vi "Teleop.vi"(10 "Match Info":T3={"Autonomous Elapsed Seconds"=0.0, "TeleOp Elapsed Seconds"=0.0, "Disabled Elapsed Seconds"=0.0, "Visited Autonomous"=FALSE, "Visited TeleOp"=FALSE, "Visited Disabled"=FALSE, "Autonomous Settings"={"Autonomous Style"=enum."Independent", "VI Refnum"=refnum}}, 11 "Call Context":T4) -> ()   [LabVIEW 2020]
doc: "This VI is called for each TeleOp packet received from the DS where the robot is not disabled. It is often used to read from the joysticks and update I/O or to update setpoints for timed control loops. It should complete and return within 20 milliseconds or it may miss DS packets."
uses:
  <vilib>/Rock Robotics/WPI/DriverStation/WPI_DriverStationDerivedRobotMode.ctl
  <vilib>/Rock Robotics/WPI/DriverStation/WPI_DriverStationMatch Info.ctl
  <vilib>/Rock Robotics/WPI/ThirdParty/Phoenix-LabVIEW/Motor Controller/Controls/CTRE_Phoenix_MotorControl_ControlMode.ctl
  <vilib>/Rock Robotics/WPI/Utilities/WPI_GetSetVariantRefNum.vi
  <vilib>/Rock Robotics/Network Tables/NT Write Boolean Array.vi
  <vilib>/Rock Robotics/Network Tables/NT Write Numeric Array.vi
  <vilib>/Rock Robotics/WPI/ThirdParty/Phoenix-LabVIEW/Motor Controller/Get/CTRE_Phoenix_MotorController_GetSelectedSensorData.vi
  <vilib>/Rock Robotics/WPI/ThirdParty/Phoenix-LabVIEW/Motor Controller/Get/CTRE_Phoenix_MotorController_GetSupplyAndStatorCurrent_Enhanced.vi
  TitanLib/Lib/TitanLib.lvlib
panel:
  in  "I Zone":dbl=1000.0
  in  "F":dbl=0.0461
  in  "D":dbl
  in  "I":dbl=0.001
  in  "P":dbl=0.1
  in  "Set PIDF":bool=TRUE
  in  "Setpoint":dbl=7000.0
  out "Current":T1(graph)
  out "PID Output":T2(graph)
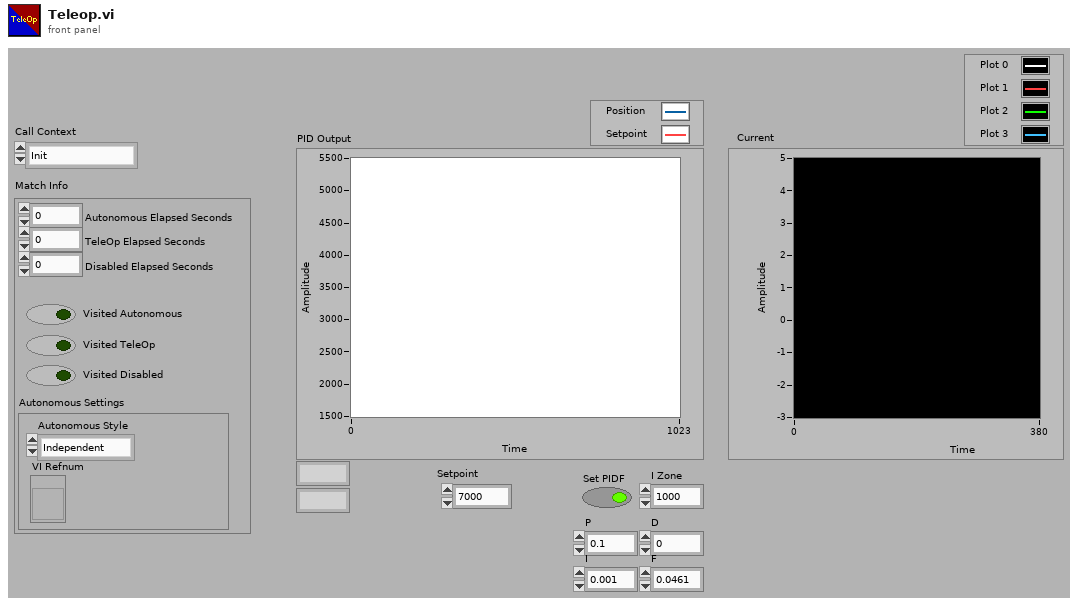
[diagram p1: front panel]
types:
  T1 = cluster{"Supply Current":dbl, "Stator Current":dbl}
  T2 = cluster{"Setpoint Position":dbl, "Position (Raw Sensor Units)":i32}
  T3 = typedef "WPI_DriverStationMatch Info.ctl" = cluster{"Autonomous Elapsed Seconds":dbl, "TeleOp Elapsed Seconds":dbl, "Disabled Elapsed Seconds":dbl, "Visited Autonomous":bool, "Visited TeleOp":bool, "Visited Disabled":bool, "Autonomous Settings":cluster{"Autonomous Style":enum16{"Iterative", "Independent"}, "VI Refnum":refnum<vi>}}
  T4 = typedef "WPI_DriverStationDerivedRobotMode.ctl" = enum16{"Init", "Execute", "Stop"}
  T5 = typedef "WPI_JoystickDevRef.ctl" = cluster{"Device":T6}
  T6 = typedef "WPI_JoystickDeviceEnum.ctl" = enum16{"USB 0", "USB 1", "USB 2", "USB 3", "USB 4", "USB 5"}
  T7 = typedef "WPI_MotorControlDeviceRef.ctl" = cluster{"DeviceStatus":errorcluster, "Type":T8, "PWM":cluster{"PWM Channel":T9, "DeadBand":T10}, "CAN":cluster{"Device Number":u8, "SetOutput VI Ref":variant, "GetOutput VI Ref":variant, "Enable VI Ref":variant, "Disable VI Ref":variant, "Data":variant}, "Invert":bool, "DIO PWM":cluster{"PWM \"Enable\" Channel":T9, "DIOChannel":T11, "PWM Rate":dbl}}
  T8 = typedef "WPI_MotorControlType.ctl" = enum16{"PWM", "CAN", "DIO PWM"}
  T9 = typedef "FPGA_DIOPWMChannel.ctl" = enum8{"PWM 0", "PWM 1", "PWM 2", "PWM 3", "PWM 4", "PWM 5", "PWM 6", "PWM 7", "PWM 8", "PWM 9", "PWM MXP 0", "PWM MXP 1", "PWM MXP 2", "PWM MXP 3", "PWM MXP 4", "PWM MXP 5", "PWM MXP 6", "PWM MXP 7", "PWM MXP 8", "PWM MXP 9", "Invalid"}
  T10 = typedef "WPI_PWMDeadband.ctl" = cluster{"Name":string, "maxPositivePwm":i32, "minPositivePwm":i32, "centerPwm":i32, "maxNegativePwm":i32, "minNegativePwm":i32, "angularRange":u16}
  T11 = typedef "FPGA_DIOChannel.ctl" = enum8{"DIO 0", "DIO 1", "DIO 2", "DIO 3", "DIO 4", "DIO 5", "DIO 6", "DIO 7", "DIO 8", "DIO 9", "DIO MXP 0", "DIO MXP 1", "DIO MXP 2", "DIO MXP 3", "DIO MXP 4", "DIO MXP 5", "DIO MXP 6", "DIO MXP 7", "DIO MXP 8", "DIO MXP 9", "DIO MXP 10", "DIO MXP 11", "DIO MXP 12", "DIO MXP 13", "DIO MXP 14", "DIO MXP 15", "SPI Port CS1", "SPI Port CS2", "SPI Port CS3", "SPI Port MISO", "SPI Port MOSI", "Invalid"}
  T12 = typedef "CTRE_Phoenix_MotorControl_ControlMode.ctl" = u16
  T13 = cluster{"Setpoint":dbl, "Position (Raw Sensor Units)":i32}
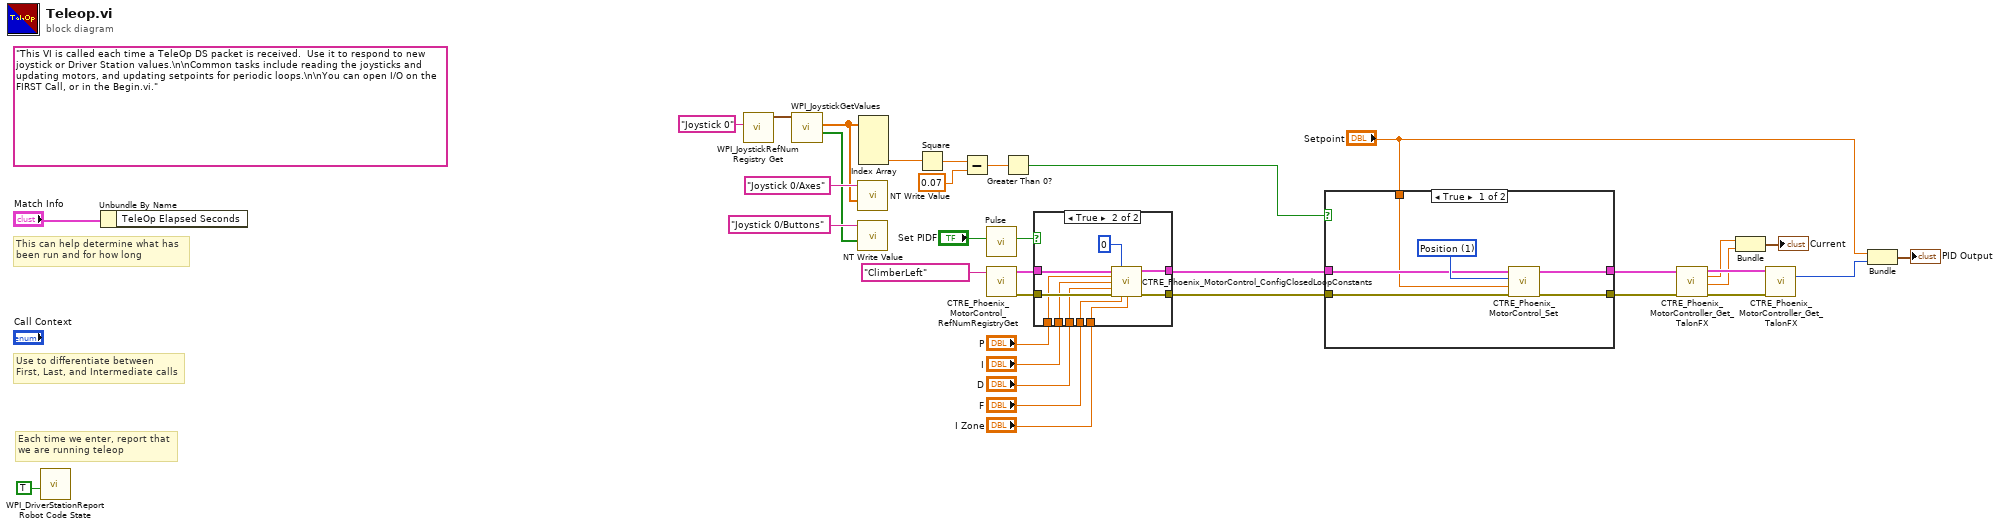
[diagram p0: block diagram]
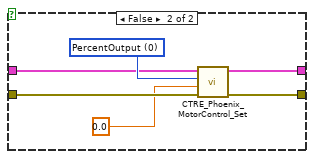
[diagram p2: hidden frame]
diagram:
  (unwired) "This VI is called each time a TeleOp DS packet is received.  Use it to respond to new joystick or Driver Station values.\n\nCommon tasks include reading the joysticks and updating motors, and updating setpoints for periodic loops.\n\nYou can open I/O on the FIRST Call, or in the Begin.vi."
  # "Each time we enter, report that\nwe are running teleop"
  # "Use to differentiate between\nFirst, Last, and Intermediate calls"
  # "This can help determine what has\nbeen run and for how long"
  n1 = call <vilib>:"WPI_DriverStationReport Robot Code State.vi"("TeleOp"=TRUE ("Autonomous")) -> ()  [unwired: 10 in, 1 out]
  n2 = Unbundle By Name("Match Info") -> ()  [unwired: 1 out]
  n3 = call <vilib>:"WPI_JoystickRefNum Registry Get.vi"("refnum name"="Joystick 0") -> ("JoystickDevRef"=w33:T5)  [unwired: 1 in, 9 out]
  n4 = call <vilib>:"WPI_JoystickGetValues.vi"("JoystickDevRef"=w33) -> ("Buttons"=w10:bool[], "Axes"=w29:dbl[])  [unwired: 6 in, 3 out]
  n5 = call-poly <vilib>:"NT Write Value.vi"("Numeric Array"=w29, "Name"="Joystick 0/Axes") -> ()  [unwired: 9 in, 1 out]
  n6 = call-poly <vilib>:"NT Write Value.vi"("Boolean Array"=w10, "Name"="Joystick 0/Buttons") -> ()  [unwired: 9 in, 1 out]
  n7 = Index Array(array=w29) -> (element #4=w4:dbl)  [unwired: 4 in, 3 out]
  n8 = Square(x=w4) -> (x^2=w8:dbl)
  n9 = Subtract(x=w8, y=0.07) -> (x-y=w6:dbl)
  n10 = call "Pulse.vi"("Input"="Set PIDF") -> ("Output"=w20:bool)  [unwired: 10 in]
  n11 = call <vilib>:"CTRE_Phoenix_MotorControl_RefNumRegistryGet.vi"("refnum name"="ClimberLeft") -> ("error out"=w22:errorcluster, "PhoenixMotorControlDevRef"=w23:T7)  [unwired: 9 in]
  n12 = Greater Than 0?(x=w6) -> (x > 0?=w1:bool)
  n13 = case shown="True" w20 {
    tunnel: w23 -> [w37 w47]
    tunnel: w22 -> [w36 w46]
    tunnel: "P" -> [_ w45]
    tunnel: "I" -> [_ w44]
    tunnel: "D" -> [_ w43]
    tunnel: "F" -> [_ w42]
    tunnel: [w37 w40] -> w12
    tunnel: [w36 w39] -> w11
    tunnel: "I Zone" -> [_ w38]
    frame False {
    }
    frame True {
      n14 = call <vilib>:"CTRE_Phoenix_MotorControl_ConfigClosedLoopConstants.vi"("PhoenixMotorControlDevRef"=w47, "slotIdx"=0, "P"=w45, "I"=w44, "D"=w43, "error in (no error)"=w46, "F"=w42, "I Zone"=w38) -> ("PhoenixMotorControlDevRef"=w40:T7, "error out"=w39:errorcluster)  [unwired: 6 in]
    }
  }
  n15 = case shown="True" w1 {
    tunnel: [w52 w58] -> w15
    tunnel: [w51 w57] -> w14
    tunnel: w12 -> [w50 w54]
    tunnel: w11 -> [w49 w56]
    tunnel: "Setpoint" -> [w48 _]
    frame True {
      w53 = T12 1 items=["PercentOutput"=0, "Position"=1, "Velocity"=2, "Current"=3, "Follower"=5, "MotionProfile"=6, "MotionMagic"=7, "MotionProfileArc"=10, "Disabled"=15] ("Control Mode")
      n16 = call <vilib>:"CTRE_Phoenix_MotorControl_Set.vi"("error in (no error)"=w49, "Output"=w48, "Control Mode"=w53, "PhoenixMotorControlDevRef"=w50) -> ("error out"=w51:errorcluster, "PhoenixMotorControlDevRef"=w52:T7)  [unwired: 6 in]
    }
    frame False {
      w59 = T12 0 items=["PercentOutput"=0, "Position"=1, "Velocity"=2, "Current"=3, "Follower"=5, "MotionProfile"=6, "MotionMagic"=7, "MotionProfileArc"=10, "Disabled"=15] ("Control Mode")
      n17 = call <vilib>:"CTRE_Phoenix_MotorControl_Set.vi"("error in (no error)"=w56, "Output"=0.0, "Control Mode"=w59, "PhoenixMotorControlDevRef"=w54) -> ("error out"=w57:errorcluster, "PhoenixMotorControlDevRef"=w58:T7)  [unwired: 6 in]
    }
  }
  n18 = call-poly <vilib>:"CTRE_Phoenix_MotorController_Get_TalonFX.vi"("PhoenixMotorControlDevRef"=w15, "error in"=w14) -> ("PhoenixMotorControlDevRef"=w27:T7, "Supply Current"=w25:dbl, "Stator Current"=w24:dbl, "error out"=w26:errorcluster)  [unwired: 10 in]
  n19 = Bundle("Supply Current"=w25, "Stator Current"=w24) -> (→"Current":T1)  [unwired: 1 in]
  n20 = call-poly <vilib>:"CTRE_Phoenix_MotorController_Get_TalonFX.vi"("PhoenixMotorControlDevRef"=w27, "error in"=w26) -> ("Position (Raw Sensor Units)"=w3:i32)  [unwired: 10 in, 3 out]
  n21 = Bundle("Setpoint"="Setpoint", "Position (Raw Sensor Units)"=w3) -> (→"PID Output":T13)  [unwired: 1 in]
